vi "setTimeLength.vi"(8 "error in (no error)":errorcluster, 10 "timeLength":dbl, 11 "PlayFile in":refnum<class "PlayFile.lvclass">) -> (0 "error out":errorcluster, 3 "PlayFile out":refnum<class "PlayFile.lvclass">)   [LabVIEW 2011, in "Tools.lvlib" / "Scripting.lvlib" / "PlayFile.lvclass"]
uses:
  PlayFile.lvclass
  PlayFile.lvclass/PlayFile.ctl
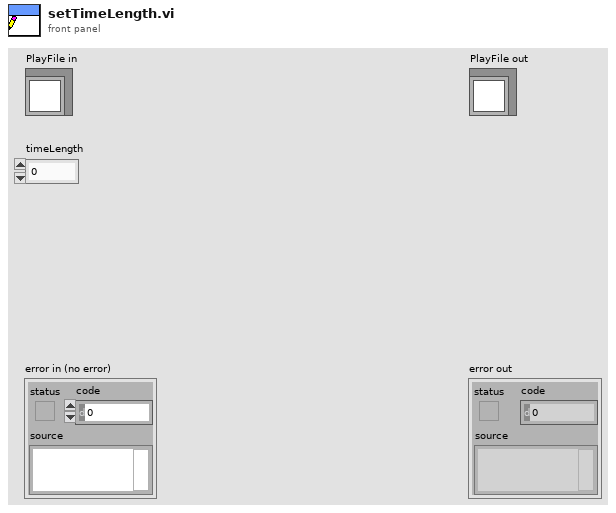
[diagram p1: front panel]
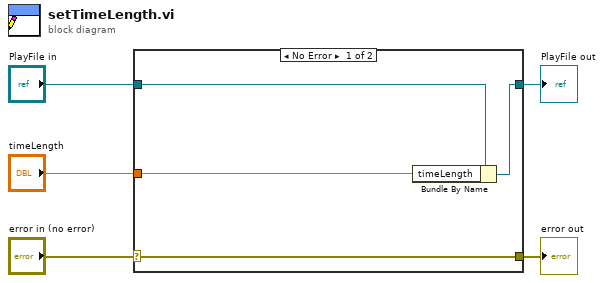
[diagram p0: block diagram]
diagram:
  n1 = case shown="No Error" "error in (no error)" {
    selector: "error in (no error)" -> [w9 w10]
    tunnel: [w9 w10] -> w4
    tunnel: [w7 w11] -> w2
    tunnel: "PlayFile in" -> [w8 w11]
    tunnel: "timeLength" -> [w6 _]
    frame No Error {
      n2 = Bundle By Name(cluster=w8, "timeLength"=w6) -> (w7:refnum<class "PlayFile.lvclass">)
    }
    frame Error {
    }
  }
  "error out" <- w4
  "PlayFile out" <- w2
